vi "Create New Directories from single path.vi"(0 "Create Directory Path":path, 11 "error in":errorcluster) -> (15 "error out":errorcluster)   [LabVIEW 2011]
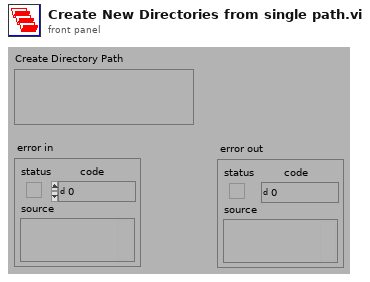
[diagram p1: front panel]
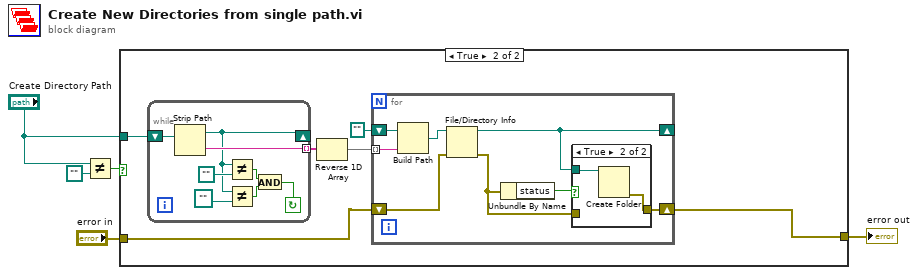
[diagram p0: block diagram]
diagram:
  n1 = Not Equal?(x="Create Directory Path", y=path "") -> (x != y?=w3:bool)
  n2 = case shown="True" w3 {
    tunnel: "Create Directory Path" -> [_ w12]
    tunnel: "error in" -> [w6 w8]
    tunnel: [w6 w7] -> w1
    frame False {
    }
    frame True {
      n3 = while {
        shift-left: w12 -> [w20]
        shift-right: [w17] -> _
        tunnel: [w19] -> w11 mode=indexing
        stop <- w13 continue-if-true
        n4 = Strip Path(path=w20) -> (stripped path=w17:path, name=w19:string)
        n5 = Not Equal?(x=w17, y=path "") -> (x != y?=w15:bool)
        n6 = Not Equal?(x=w17, y=path "") -> (x != y?=w14:bool)
        n7 = And(x=w15, y=w14) -> (x .and. y?=w13:bool)
      }
      n8 = Reverse 1D Array(array=w11) -> (reversed array=w10:string[])
      n9 = for {
        tunnel: w10 -> [w27] mode=indexing
        shift-right: [w24] -> _
        shift-left: path "" -> [w28]
        shift-right: [w22] -> w7
        shift-left: w8 -> [w21]
        n10 = Build Path(base path=w28, name or relative path=w27) -> (appended path=w25:path)
        n11 = File/Directory Info(path=w25, error in=w21) -> (path out=w24:path, error out=w23:errorcluster)  [unwired: 5 out]
        n12 = Unbundle By Name(w23) -> ("status"=w26:bool)
        n13 = case shown="True" w26 {
          tunnel: w24 -> [_ w31]
          tunnel: w23 -> [w29 _]
          tunnel: [w29 w30] -> w22
          frame False {
          }
          frame True {
            n14 = Create Folder(path (use dialog)=w31) -> (error out=w30:errorcluster)  [unwired: 2 in, 2 out]
          }
        }
      }
    }
  }
  "error out" <- w1
